vi "平行样启动流程对话框.vi"() -> (1 "启动模块":T1, 2 "常规启动":bool, 3 "确定启动":bool)   [LabVIEW 2016, in "质控单元.lvlib"]
uses:
  <vilib>/Utility/miscctls.llb/LVPointTypeDef.ctl
panel:
  in  "直接启动":bool
  in  "取消":bool
  in  "常规启动":bool
  # "请选择启动模式"
  # "常规启动：先启动采配水，再进行平行样测试"
  # "直接启动：不启动采配水，直接平行样测试"
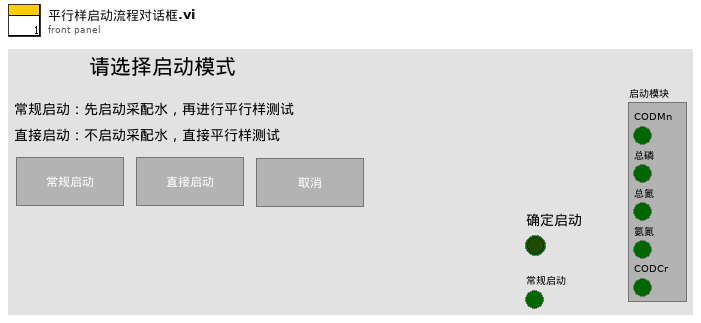
[diagram p1: front panel]
types:
  T1 = cluster{"CODMn":bool, "总磷":bool, "总氮":bool, "氨氮":bool, "CODCr":bool}
  T2 = typedef "LVPointTypeDef.ctl" = cluster{"Horizontal":i16, "Vertical":i16}
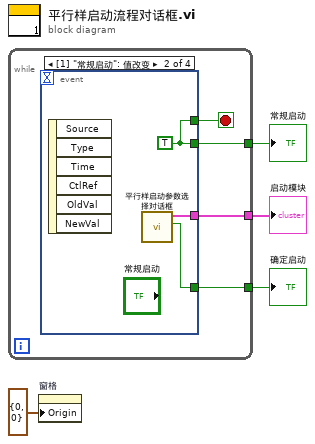
[diagram p0: block diagram]
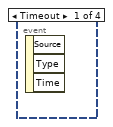
[diagram p2: hidden frame]
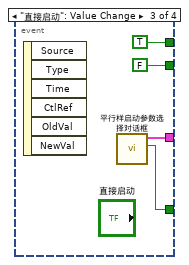
[diagram p3: hidden frame]
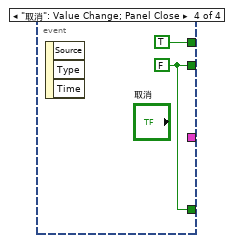
[diagram p4: hidden frame]
diagram:
  n1 = while {
    tunnel: [w7] -> w4
    tunnel: [w6] -> w2
    tunnel: [w5] -> w3
    stop <- w8 stop-if-true
    n2 = event shown="[1] \"常规启动\": 值改变" {
      selector: _ -> [_ _ _ _]
      dyn-events: _ -> [_ _ _ _]
      timeout: _ -> [_ _ _ _]
      tunnel: [_ w11 TRUE ("确定") TRUE ("确定")] -> w8
      tunnel: [_ w11 FALSE ("确定") w16] -> w7
      tunnel: [_ w10 w13 _] -> w6
      tunnel: [_ w9 w12 w16] -> w5
      event Timeout {
        n3 = event-data() -> ()  [unwired: 1 in, 3 out]
      }
      event "常规启动": Value Change {
        w11 = TRUE ("确定")
        n4 = event-data() -> ()  [unwired: 1 in, 6 out]
        n5 = call "平行样启动参数选择对话框.vi"() -> ("确定启动"=w9:bool, "启动模块"=w10:T1)  [unwired: 10 in]
      }
      event "直接启动": Value Change {
        n6 = event-data() -> ()  [unwired: 1 in, 6 out]
        n7 = call "平行样启动参数选择对话框.vi"() -> ("确定启动"=w12:bool, "启动模块"=w13:T1)  [unwired: 10 in]
      }
      event "取消": Value Change; Panel Close {
        w16 = FALSE ("确定")
        n8 = event-data() -> ()  [unwired: 1 in, 3 out]
      }
    }
  }
  "常规启动" <- w4
  "确定启动" <- w3
  "启动模块" <- w2
  n9 = property on="窗格" class="Pane"("Origin"=T2 {"Horizontal"=0, "Vertical"=0} ("原点")) -> ()  [unwired: 2 in, 2 out]
